vi "First.vi"(0 "object in":refnum<class "DFSTreeIterator.lvclass">, 5 "Error In":errorcluster) -> (14 "object out":refnum<class "DFSTreeIterator.lvclass">, 16 "Root":refnum<class "Node.lvclass">, 19 "Error Out":errorcluster)   [LabVIEW 2024, in "DFSTreeIterator.lvclass"]
doc: "Returns root of the collection"
uses:
  DFSTreeIterator.lvclass
  Node_class/Node.lvclass
  DFSTreeIterator.lvclass/DFSTreeIterator.ctl
  Tree_class/Tree.lvclass
panel:
  # "Connector Pane"
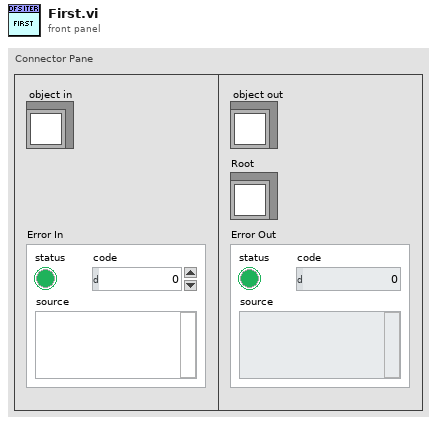
[diagram p1: front panel]
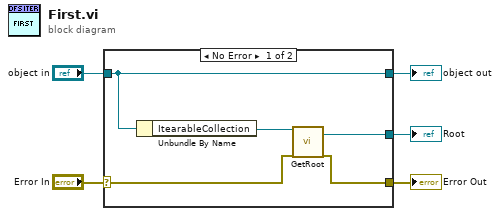
[diagram p0: block diagram]
diagram:
  n1 = case shown="No Error" "Error In" {
    selector: "Error In" -> [w8 w12]
    tunnel: [w7 w12] -> w4
    tunnel: [w10 w11] -> w2
    tunnel: "object in" -> [w10 w11]
    tunnel: [w6 _] -> w1
    frame No Error {
      n2 = Unbundle By Name(w10) -> ("ItearableCollection"=w9:refnum<class "Tree.lvclass">)
      n3 = call-dynamic "GetRoot.vi"("object in"=w9, "Error In"=w8) -> ("Root"=w6:refnum<class "Node.lvclass">, "Error Out"=w7:errorcluster)  [unwired: 15 in, 1 out]
    }
    frame Error {
    }
  }
  "Error Out" <- w4
  "object out" <- w2
  "Root" <- w1
